vi "pcbDryRunPrep.vi"() -> ()   [LabVIEW 2015]
uses:
  GlobalPath.vi
  GlobalData.vi
  GlobalVi.vi
panel:
  in  "visual 9":bool caption="Switch on the table vacuum"
  in  "visual 8":bool caption="Wait 24h for the glue to cure"
  in  "visual 7":bool caption="Glue the interconnections"
  in  "visual 6":bool caption="Check the cleanliness of the interconnections"
  in  "visual 5":bool caption="Remove the table vacuum"
  in  "visual 4":bool caption="Add kapton strips (thickness 60x2) under the frame and cooling bar region to lift them"
  in  "visual 3":bool caption="Close cut outs using kapton and the metallic pieces removed in the beginning"
  in  "DONE ALL?":bool
  out "appended path":path
  out "PanelName":string
  in  "rasnik program":bool
  in  "Done?":bool
  in  "visual 2":bool caption="Cover all PCB holes with kapton apart from the (PCB/Cooling bar/frame) positioning holes"
  # "1. Interconnection gluing"
  # "2. PCB glue protection"
  # "3. Rasnik mask reading from C-CCDs (final reading before gluing)"
  # "The PCB on the table/stiffback will be read through the appropriate vi program"
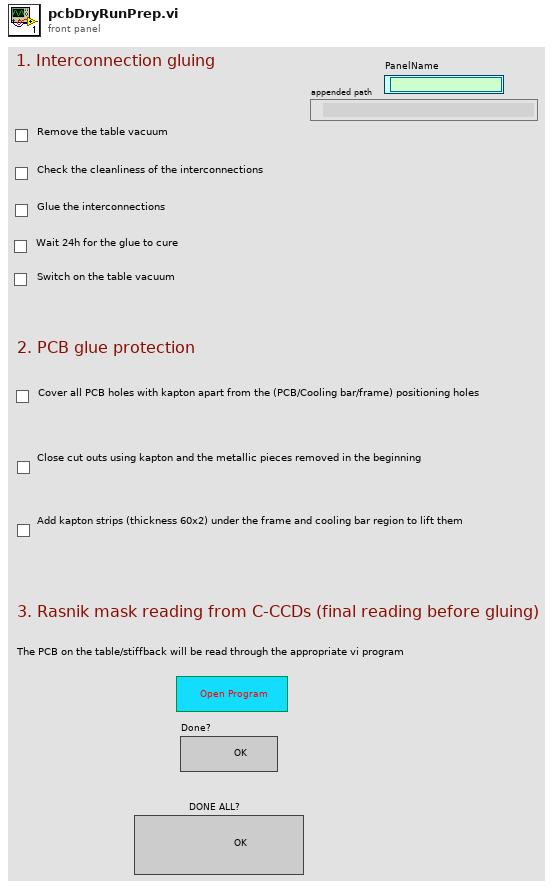
[diagram p1: front panel]
types:
  T1 = enum16{"open", "replace", "create", "open or create", "replace or create", "replace or create with confirmation"}
  T2 = enum32{"Bad", "Idle", "Run top level", "Running"}
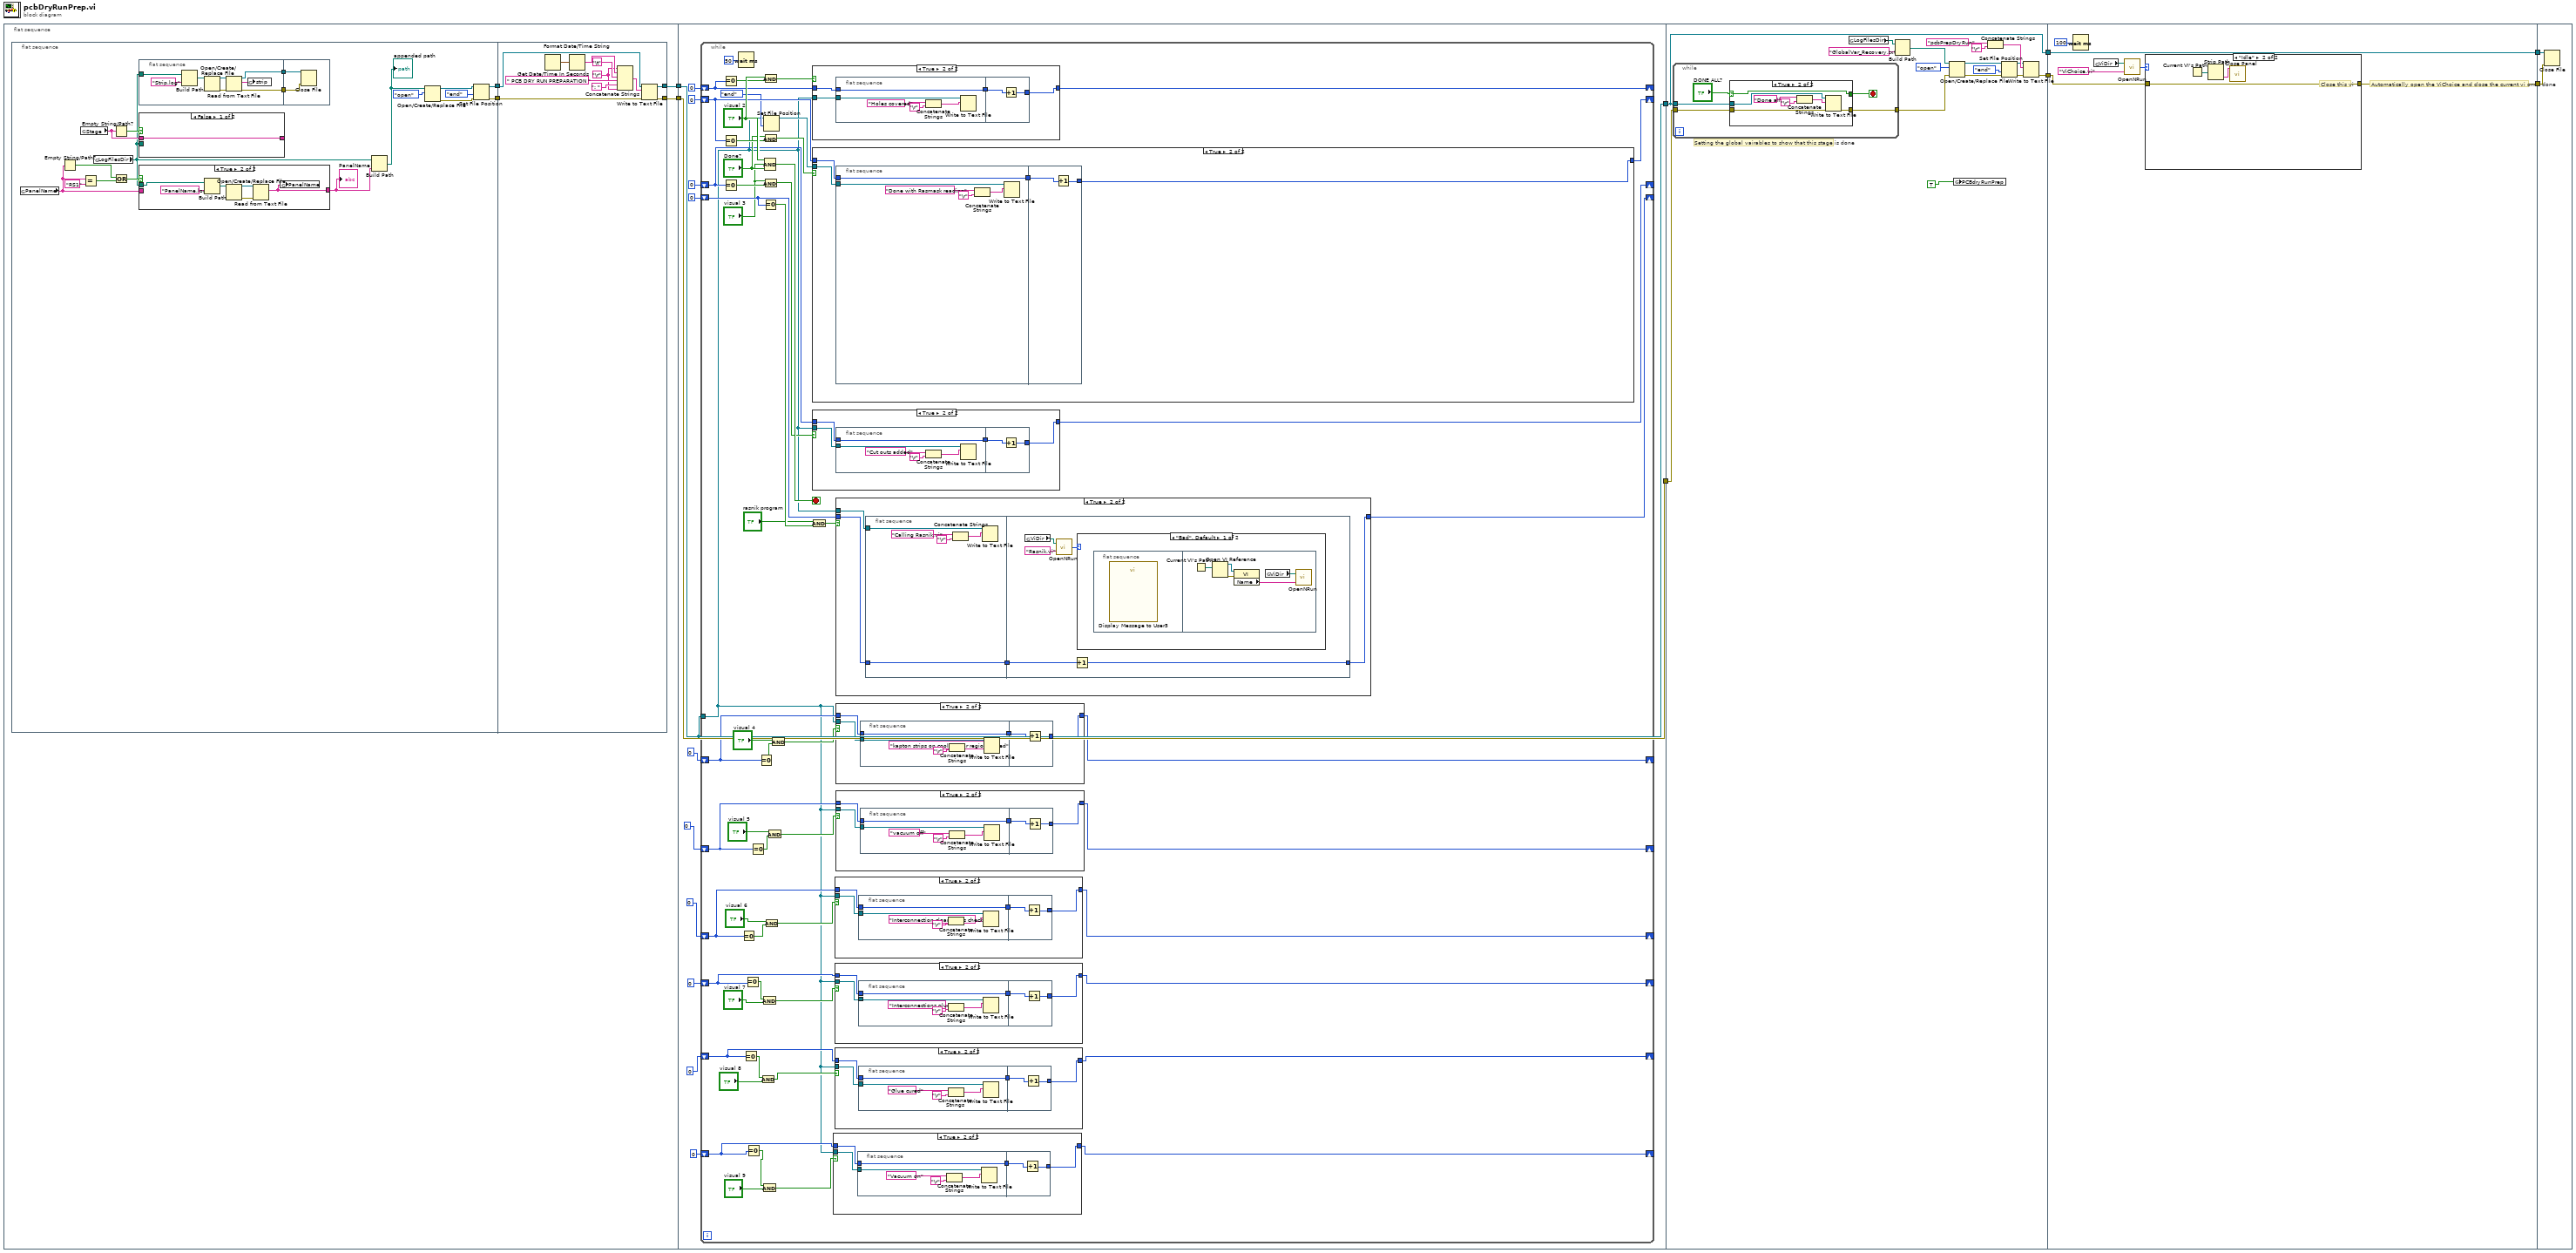
[diagram p0: block diagram]
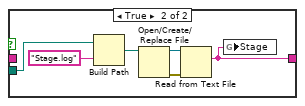
[diagram p2: hidden frame]
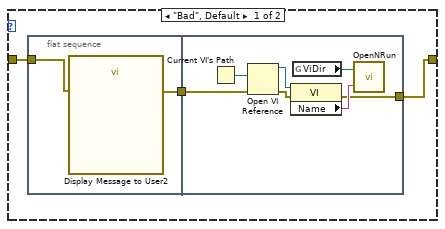
[diagram p16: hidden frame]
diagram:
  n1 = flat-sequence {
    tunnel: [w11] -> w8
    tunnel: [w10] -> w7
    tunnel: w8 -> [w77]
    tunnel: w7 -> [w66]
    tunnel: [w77] -> w2
    tunnel: [w66] -> w1
    tunnel: w2 -> [w264]
    tunnel: [w264] -> w6
    tunnel: [w267] -> w4
    tunnel: w1 -> [w262]
    tunnel: w6 -> [w298]
    tunnel: [w298] -> w5
    tunnel: w4 -> [w294]
    tunnel: [w293] -> w3
    tunnel: w5 -> [w314]
    tunnel: w3 -> [w315]
    frame #0 {
      n2 = flat-sequence {
        tunnel: [w25] -> w12
        tunnel: [w24] -> w9
        tunnel: w12 -> [w61]
        tunnel: [w60] -> w11
        tunnel: [w59] -> w10
        tunnel: w9 -> [w58]
        frame #0 {
          n3 = global read "GlobalData.vi" "PanelName"() -> (w18:string)
          n4 = Empty String/Path?(string/path=w18) -> (empty?=w20:bool)
          n5 = global read "GlobalData.vi" "Stage"() -> (w22:string)
          n6 = Equal?(x=w18, y="RS1") -> (x = y?=w16:bool)
          n7 = global read "GlobalPath.vi" "LogFilesDir"() -> (w13:path)
          n8 = Empty String/Path?(string/path=w22) -> (empty?=w23:bool)
          n9 = Or(x=w20, y=w16) -> (x .or. y?=w19:bool)
          n10 = flat-sequence {
            tunnel: w13 -> [w38]
            tunnel: [w32] -> w15
            tunnel: [w31] -> w14
            tunnel: w15 -> [w40]
            tunnel: w14 -> [w39]
            frame #0 {
              n11 = Build Path(base path=w38, name or relative path="Strip.log") -> (appended path=w37:path)
              n12 = Open/Create/Replace File(file path (use dialog)=w37) -> (refnum out=w34:refnum<file>, error out=w35:errorcluster)  [unwired: 5 in, 1 out]
              n13 = Read from Text File(file (use dialog)=w34, error in=w35) -> (refnum out=w31:refnum<file>, text=w33:string, error out=w32:errorcluster)  [unwired: 2 in, 1 out]
              n14 = global write "GlobalData.vi" "strip"(w33) -> ()
            }
            frame #1 {
              n15 = Close File(refnum=w39, error in=w40) -> ()  [unwired: 2 out]
            }
          }
          n16 = case shown="False" w23 {
            tunnel: w13 -> [_ w47]
            tunnel: [w41 w42] -> _
            tunnel: w22 -> [w41 _]
            frame False {
            }
            frame True {
              n17 = Build Path(base path=w47, name or relative path="Stage.log") -> (appended path=w46:path)
              n18 = Open/Create/Replace File(file path (use dialog)=w46) -> (refnum out=w43:refnum<file>, error out=w44:errorcluster)  [unwired: 5 in, 1 out]
              n19 = Read from Text File(file (use dialog)=w43, error in=w44) -> (text=w42:string)  [unwired: 2 in, 3 out]
              n20 = global write "GlobalData.vi" "Stage"(w42) -> ()
            }
          }
          n21 = case shown="True" w19 {
            tunnel: w13 -> [_ w54]
            tunnel: [w48 w49] -> w21
            tunnel: w18 -> [w48 _]
            frame False {
            }
            frame True {
              n22 = Build Path(base path=w54, name or relative path="PanelName.log") -> (appended path=w53:path)
              n23 = Open/Create/Replace File(file path (use dialog)=w53) -> (refnum out=w50:refnum<file>, error out=w51:errorcluster)  [unwired: 5 in, 1 out]
              n24 = Read from Text File(file (use dialog)=w50, error in=w51) -> (text=w49:string)  [unwired: 2 in, 3 out]
              n25 = global write "GlobalData.vi" "PanelName"(w49) -> ()
            }
          }
          "PanelName" <- w21
          n26 = Build Path(base path=w13, name or relative path=w21) -> (appended path=w30:path)
          "appended path" <- w30
          n27 = Open/Create/Replace File(file path (use dialog)=w30, operation (0:open)=T1."open") -> (refnum out=w27:refnum<file>, error out=w26:errorcluster)  [unwired: 4 in, 1 out]
          n28 = Set File Position(refnum=w27, from (0:start)=enum16{"start", "end", "current"}."end", error in=w26) -> (refnum out=w25:refnum<file>, error out=w24:errorcluster)  [unwired: 1 in]
        }
        frame #1 {
          w55 = "\r"
          n29 = Get Date/Time In Seconds() -> (seconds since 1Jan1904=w57:timestamp)
          n30 = Format Date/Time String(seconds (now)=w57) -> (date/time string=w63:string)  [unwired: 2 in]
          n31 = Concatenate Strings(w55, w63, "\t", " PCB DRY RUN PREPARATION ", ": ", w55) -> (w62:string)
          n32 = Write to Text File(file (use dialog)=w61, text=w62, error in=w58) -> (refnum out=w60:refnum<file>, error out=w59:errorcluster)  [unwired: 1 in, 1 out]
        }
      }
    }
    frame #1 {
      n33 = while {
        tunnel: w77 -> [w84]
        shift-right: [w131] -> _
        shift-left: 0 -> [w129]
        shift-right: [w122] -> _
        shift-left: 0 -> [w123]
        shift-right: [w117] -> _
        shift-left: 0 -> [w118]
        shift-right: [w110] -> _
        shift-left: 0 -> [w111]
        shift-right: [w78] -> _
        shift-left: 0 -> [w90]
        shift-right: [w79] -> _
        shift-left: 0 -> [w89]
        shift-right: [w80] -> _
        shift-left: 0 -> [w88]
        shift-right: [w81] -> _
        shift-left: 0 -> [w87]
        shift-right: [w82] -> _
        shift-left: 0 -> [w86]
        shift-right: [w83] -> _
        shift-left: 0 -> [w85]
        stop <- w114 stop-if-true
        n34 = Equal To 0?(x=w129) -> (x = 0?=w128:bool)
        n35 = Equal To 0?(x=w118) -> (x = 0?=w121:bool)
        n36 = Equal To 0?(x=w111) -> (x = 0?=w113:bool)
        n37 = Wait (ms)(milliseconds to wait=u32 50) -> ()  [unwired: 1 out]
        n38 = Equal To 0?(x=w88) -> (x = 0?=w95:bool)
        n39 = Equal To 0?(x=w86) -> (x = 0?=w102:bool)
        n40 = Equal To 0?(x=w87) -> (x = 0?=w99:bool)
        n41 = Equal To 0?(x=w85) -> (x = 0?=w105:bool)
        n42 = Equal To 0?(x=w89) -> (x = 0?=w93:bool)
        n43 = Equal To 0?(x=w90) -> (x = 0?=w107:bool)
        n44 = And(x=w102, y="visual 8") -> (x .and. y?=w100:bool)
        n45 = And(x=w99, y="visual 7") -> (x .and. y?=w97:bool)
        n46 = And(x=w105, y="visual 9") -> (x .and. y?=w103:bool)
        n47 = And(x="visual 2", y=w128) -> (x .and. y?=w127:bool)
        n48 = And(x="Done?", y=w121) -> (x .and. y?=w119:bool)
        n49 = And(x="visual 3", y=w113) -> (x .and. y?=w112:bool)
        n50 = Equal To 0?(x=w123) -> (x = 0?=w126:bool)
        n51 = Set File Position(refnum=w84, from (0:start)=enum16{"start", "end", "current"}."end") -> (refnum out=w115:refnum<file>)  [unwired: 2 in, 1 out]
        n52 = And(x="visual 6", y=w95) -> (x .and. y?=w94:bool)
        n53 = Compound Arithmetic op=AND("visual 2", "visual 3", "Done?") -> (w114:bool)
        n54 = And(x="visual 5", y=w93) -> (x .and. y?=w91:bool)
        n55 = And(x="visual 4", y=w107) -> (x .and. y?=w106:bool)
        n56 = And(x="rasnik program", y=w126) -> (x .and. y?=w124:bool)
        n57 = case shown="True" w127 {
          tunnel: w84 -> [_ w253]
          tunnel: w129 -> [w249 w252]
          tunnel: [w249 w250] -> w131
          frame False {
          }
          frame True {
            n58 = flat-sequence {
              tunnel: w253 -> [w255]
              tunnel: w252 -> [w254]
              tunnel: [w254] -> w251
              tunnel: w251 -> [w260]
              tunnel: [w259] -> w250
              frame #0 {
                n59 = Concatenate Strings("Holes covered", "\r") -> (w258:string)
                n60 = Write to Text File(file (use dialog)=w255, text=w258) -> ()  [unwired: 2 in, 3 out]
              }
              frame #1 {
                n61 = Increment(x=w260) -> (x+1=w259:i32)
              }
            }
          }
        }
        n62 = case shown="True" w119 {
          tunnel: w115 -> [_ w220]
          tunnel: [w217 w219] -> w117
          tunnel: w118 -> [w217 w218]
          frame False {
          }
          frame True {
            n63 = flat-sequence {
              tunnel: w220 -> [w223]
              tunnel: [w222] -> w221
              tunnel: w218 -> [w222]
              tunnel: w221 -> [w227]
              tunnel: [w228] -> w219
              frame #0 {
                n64 = Concatenate Strings("Done with Rasmask reading", "\r") -> (w226:string)
                n65 = Write to Text File(file (use dialog)=w223, text=w226) -> ()  [unwired: 2 in, 3 out]
              }
              frame #1 {
                n66 = Increment(x=w227) -> (x+1=w228:i32)
              }
            }
          }
        }
        n67 = case shown="True" w112 {
          tunnel: w111 -> [w205 w209]
          tunnel: [w205 w207] -> w110
          tunnel: w84 -> [_ w206]
          frame False {
          }
          frame True {
            n68 = flat-sequence {
              tunnel: w206 -> [w211]
              tunnel: w209 -> [w210]
              tunnel: [w210] -> w208
              tunnel: w208 -> [w216]
              tunnel: [w215] -> w207
              frame #0 {
                n69 = Concatenate Strings("Cut outs added", "\r") -> (w214:string)
                n70 = Write to Text File(file (use dialog)=w211, text=w214) -> ()  [unwired: 2 in, 3 out]
              }
              frame #1 {
                n71 = Increment(x=w216) -> (x+1=w215:i32)
              }
            }
          }
        }
        n72 = case shown="True" w103 {
          tunnel: w85 -> [w133 w137]
          tunnel: [w133 w135] -> w83
          tunnel: w84 -> [_ w134]
          frame False {
          }
          frame True {
            n73 = flat-sequence {
              tunnel: w134 -> [w139]
              tunnel: w137 -> [w138]
              tunnel: [w138] -> w136
              tunnel: w136 -> [w144]
              tunnel: [w143] -> w135
              frame #0 {
                n74 = Concatenate Strings("Vacuum on", "\r") -> (w142:string)
                n75 = Write to Text File(file (use dialog)=w139, text=w142) -> ()  [unwired: 2 in, 3 out]
              }
              frame #1 {
                n76 = Increment(x=w144) -> (x+1=w143:i32)
              }
            }
          }
        }
        n77 = case shown="True" w100 {
          tunnel: w86 -> [w145 w149]
          tunnel: [w145 w147] -> w82
          tunnel: w84 -> [_ w146]
          frame False {
          }
          frame True {
            n78 = flat-sequence {
              tunnel: w146 -> [w151]
              tunnel: w149 -> [w150]
              tunnel: [w150] -> w148
              tunnel: w148 -> [w156]
              tunnel: [w155] -> w147
              frame #0 {
                n79 = Concatenate Strings("Glue cured", "\r") -> (w154:string)
                n80 = Write to Text File(file (use dialog)=w151, text=w154) -> ()  [unwired: 2 in, 3 out]
              }
              frame #1 {
                n81 = Increment(x=w156) -> (x+1=w155:i32)
              }
            }
          }
        }
        n82 = case shown="True" w94 {
          tunnel: w88 -> [w169 w173]
          tunnel: [w169 w171] -> w80
          tunnel: w84 -> [_ w170]
          frame False {
          }
          frame True {
            n83 = flat-sequence {
              tunnel: w170 -> [w175]
              tunnel: w173 -> [w174]
              tunnel: [w174] -> w172
              tunnel: w172 -> [w180]
              tunnel: [w179] -> w171
              frame #0 {
                n84 = Concatenate Strings("Interconnection cleanliness checked", "\r") -> (w178:string)
                n85 = Write to Text File(file (use dialog)=w175, text=w178) -> ()  [unwired: 2 in, 3 out]
              }
              frame #1 {
                n86 = Increment(x=w180) -> (x+1=w179:i32)
              }
            }
          }
        }
        n87 = case shown="True" w97 {
          tunnel: w87 -> [w157 w161]
          tunnel: [w157 w159] -> w81
          tunnel: w84 -> [_ w158]
          frame False {
          }
          frame True {
            n88 = flat-sequence {
              tunnel: w158 -> [w163]
              tunnel: w161 -> [w162]
              tunnel: [w162] -> w160
              tunnel: w160 -> [w168]
              tunnel: [w167] -> w159
              frame #0 {
                n89 = Concatenate Strings("Interconnections glued", "\r") -> (w166:string)
                n90 = Write to Text File(file (use dialog)=w163, text=w166) -> ()  [unwired: 2 in, 3 out]
              }
              frame #1 {
                n91 = Increment(x=w168) -> (x+1=w167:i32)
              }
            }
          }
        }
        n92 = case shown="True" w124 {
          tunnel: w84 -> [_ w232]
          tunnel: [w229 w230] -> w122
          tunnel: w123 -> [w229 w231]
          frame False {
          }
          frame True {
            n93 = flat-sequence {
              tunnel: w232 -> [w235]
              tunnel: [w234] -> w233
              tunnel: w231 -> [w234]
              tunnel: w233 -> [w242]
              tunnel: [w243] -> w230
              frame #0 {
                n94 = Concatenate Strings("Calling Rasnik.vi", "\r") -> (w238:string)
                n95 = Write to Text File(file (use dialog)=w235, text=w238) -> ()  [unwired: 2 in, 3 out]
              }
              frame #1 {
                n96 = global read "GlobalPath.vi" "ViDir"() -> (w239:path)
                n97 = call "OpenNRun.vi"("VI name"="Rasnik.vi", "ViDirPath"=w239) -> ("Execution:State"=w240:T2)
                n98 = Increment(x=w242) -> (x+1=w243:i32)
                n99 = case shown="\"Bad\", Default" w240 {
                  frame "Bad", Default {
                    n100 = flat-sequence {
                      frame #0 {
                        n101 = call "Display Message to User3"() -> ()  [unwired: 10 in, 2 out]
                      }
                      frame #1 {
                        n102 = Current VI's Path() -> (path=w244:path)
                        n103 = Open VI Reference(vi path=w244) -> (vi reference=w248:refnum<vi>, error out=w247:errorcluster)  [unwired: 5 in]
                        n104 = property class="VI"(reference=w248, error in=w247) -> ("Name"=w245:string)  [unwired: 2 out]
                        n105 = global read "GlobalPath.vi" "ViDir"() -> (w246:path)
                        n106 = call "OpenNRun.vi"("VI name"=w245, "ViDirPath"=w246) -> ()  [unwired: 1 out]
                      }
                    }
                  }
                  frame "Idle" {
                  }
                }
              }
            }
          }
        }
        n107 = case shown="True" w106 {
          tunnel: w90 -> [w193 w197]
          tunnel: [w193 w195] -> w78
          tunnel: w84 -> [_ w194]
          frame False {
          }
          frame True {
            n108 = flat-sequence {
              tunnel: w194 -> [w199]
              tunnel: w197 -> [w198]
              tunnel: [w198] -> w196
              tunnel: w196 -> [w204]
              tunnel: [w203] -> w195
              frame #0 {
                n109 = Concatenate Strings("kapton strips on cooling bar region added", "\r") -> (w202:string)
                n110 = Write to Text File(file (use dialog)=w199, text=w202) -> ()  [unwired: 2 in, 3 out]
              }
              frame #1 {
                n111 = Increment(x=w204) -> (x+1=w203:i32)
              }
            }
          }
        }
        n112 = case shown="True" w91 {
          tunnel: w89 -> [w181 w185]
          tunnel: [w181 w183] -> w79
          tunnel: w84 -> [_ w182]
          frame False {
          }
          frame True {
            n113 = flat-sequence {
              tunnel: w182 -> [w187]
              tunnel: w185 -> [w186]
              tunnel: [w186] -> w184
              tunnel: w184 -> [w192]
              tunnel: [w191] -> w183
              frame #0 {
                n114 = Concatenate Strings("vacuum off", "\r") -> (w190:string)
                n115 = Write to Text File(file (use dialog)=w187, text=w190) -> ()  [unwired: 2 in, 3 out]
              }
              frame #1 {
                n116 = Increment(x=w192) -> (x+1=w191:i32)
              }
            }
          }
        }
      }
    }
    frame #2 {
      # "Setting the global vairables to show that this stage is done"
      n117 = while {
        tunnel: w262 -> [w281]
        tunnel: [w278] -> w265
        tunnel: w264 -> [w280]
        stop <- w279 stop-if-true
        n118 = case shown="True" "DONE ALL?" {
          selector: "DONE ALL?" -> [w284 w285]
          tunnel: [w284 w285] -> w279
          tunnel: w280 -> [_ w288]
          tunnel: w281 -> [w283 w287]
          tunnel: [w283 w286] -> w278
          frame False {
          }
          frame True {
            n119 = Concatenate Strings("Done all", "\r") -> (w291:string)
            n120 = Write to Text File(file (use dialog)=w288, text=w291, error in=w287) -> (error out=w286:errorcluster)  [unwired: 1 in, 2 out]
          }
        }
      }
      n121 = global read "GlobalPath.vi" "LogFilesDir"() -> (w266:path)
      n122 = Build Path(base path=w266, name or relative path="GlobalVar_Recovery.txt") -> (appended path=w276:path)
      n123 = Open/Create/Replace File(file path (use dialog)=w276, error in=w265, operation (0:open)=T1."open") -> (refnum out=w272:refnum<file>, error out=w273:errorcluster)  [unwired: 3 in, 1 out]
      n124 = global write "GlobalVi.vi" "PCBdryRunPrep"(TRUE) -> ()
      n125 = Concatenate Strings("pcbPrepDryRun", "\r") -> (w271:string)
      n126 = Set File Position(refnum=w272, from (0:start)=enum16{"start", "end", "current"}."end", error in=w273) -> (refnum out=w269:refnum<file>, error out=w268:errorcluster)  [unwired: 1 in]
      n127 = Write to Text File(file (use dialog)=w269, text=w271, error in=w268) -> (error out=w267:errorcluster)  [unwired: 1 in, 2 out]
    }
    frame #3 {
      # "Automatically open the ViChoice and close the current vi once done"
      n128 = Wait (ms)(milliseconds to wait=100) -> ()  [unwired: 1 out]
      n129 = global read "GlobalPath.vi" "ViDir"() -> (w297:path)
      n130 = call "OpenNRun.vi"("VI name"="ViChoice.vi", "ViDirPath"=w297) -> ("Execution:State"=w296:T2)
      n131 = case shown="\"Idle\"" w296 {
        tunnel: [w301 w311] -> w293
        tunnel: w294 -> [w299 w311]
        frame "Bad", Default {
          n132 = flat-sequence {
            tunnel: w299 -> [w303]
            tunnel: [w302] -> w300
            tunnel: [w307] -> w301
            tunnel: w300 -> [w306]
            frame #0 {
              n133 = call "Display Message to User2"("error in (no error)"=w303) -> ("error out"=w302:errorcluster)  [unwired: 9 in, 1 out]
            }
            frame #1 {
              n134 = Current VI's Path() -> (path=w304:path)
              n135 = Open VI Reference(vi path=w304, error in (no error)=w306) -> (vi reference=w310:refnum<vi>, error out=w309:errorcluster)  [unwired: 4 in]
              n136 = property class="VI"(reference=w310, error in=w309) -> (error out=w307:errorcluster, "Name"=w308:string)  [unwired: 1 out]
              n137 = global read "GlobalPath.vi" "ViDir"() -> (w305:path)
              n138 = call "OpenNRun.vi"("VI name"=w308, "ViDirPath"=w305) -> ()  [unwired: 1 out]
            }
          }
        }
        frame "Idle" {
          # "Close this vi"
          n139 = Current VI's Path() -> (path=w313:path)
          n140 = Strip Path(path=w313) -> (name=w312:string)  [unwired: 1 out]
          n141 = call <vilib>:"Close Panel.vi"("VI name"=w312) -> ()  [unwired: 10 in, 1 out]
        }
      }
    }
    frame #4 {
      n142 = Close File(refnum=w314, error in=w315) -> ()  [unwired: 2 out]
    }
  }
